vi "clLabview_BDPW_SaltFormat.vi"(9 "count Path":u32, 10 "count String":u32, 11 "count Numeric":u32) -> (3 "Salt":string)   [LabVIEW 2020, in "vi_lib.lvlib" / "clLabview.lvclass"]
uses:
  clLabview.lvclass
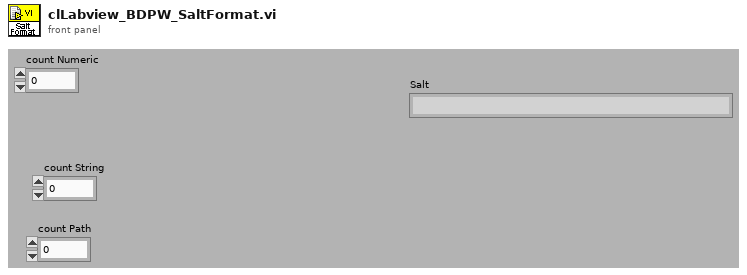
[diagram p1: front panel]
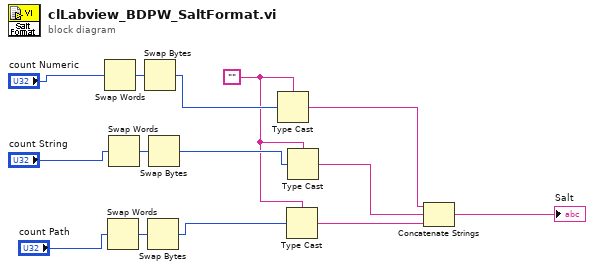
[diagram p0: block diagram]
diagram:
  w2 = "" ("MD5 message-digest 2")
  n1 = Swap Words(1:"count Numeric") -> (0:w13:u32)
  n2 = Swap Words(1:"count Path") -> (0:w5:u32)
  n3 = Swap Words(1:"count String") -> (0:w8:u32)
  n4 = Swap Bytes(anything=w13) -> (byte swapped=w12:u32)
  n5 = Swap Bytes(anything=w5) -> (byte swapped=w4:u32)
  n6 = Swap Bytes(anything=w8) -> (byte swapped=w9:u32)
  n7 = Type Cast(type=w2, x=w12) -> (*(type *) &x=w11:string)
  n8 = Type Cast(type=w2, x=w4) -> (*(type *) &x=w3:string)
  n9 = Type Cast(type=w2, x=w9) -> (*(type *) &x=w10:string)
  n10 = Concatenate Strings(w11, w10, w3) -> (→"Salt":string)
